vi "Read Static (Func Global).vi"(8 "error in (no error)":errorcluster, 11 "MementoNumeric in":refnum<class "MementoNumeric.lvclass">) -> (0 "error out":errorcluster, 2 "Static (Func Global)":i32, 3 "MementoNumeric out":refnum<class "MementoNumeric.lvclass">)   [LabVIEW 2009, in "MementoNumeric.lvclass"]
uses:
  MementoNumeric.lvclass
  MementoNumeric.lvclass/MementoNumeric.ctl
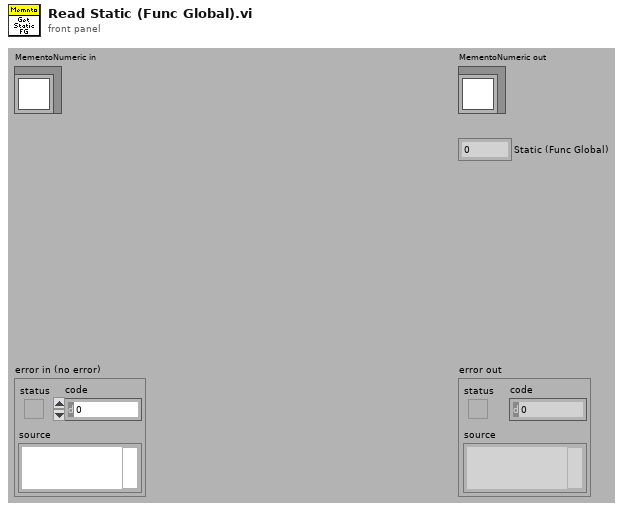
[diagram p1: front panel]
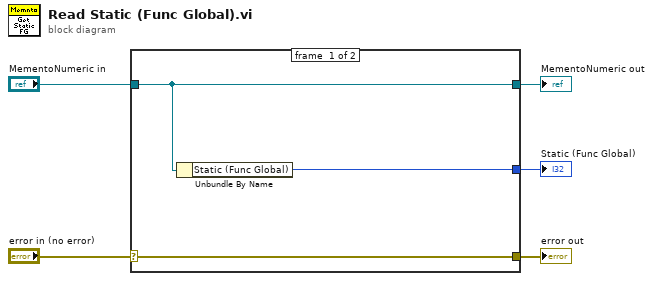
[diagram p0: block diagram]
diagram:
  n1 = case shown="No Error" "error in (no error)" {
    selector: "error in (no error)" -> [w8 w9]
    tunnel: [w8 w9] -> w4
    tunnel: [w7 w10] -> w2
    tunnel: "MementoNumeric in" -> [w7 w10]
    tunnel: [w6 _] -> w1
    frame #0 {
      n2 = Unbundle By Name(w7) -> ("Static (Func Global)"=w6:i32)
    }
    frame #1 {
    }
  }
  "error out" <- w4
  "MementoNumeric out" <- w2
  "Static (Func Global)" <- w1
